vi "LabVIEW_2_Arduino_3D_Print_Fan_Zhu.vi"() -> ()   [LabVIEW 2017]
uses:
  <vilib>/Instr/_visa.llb/VISA Flush IO Buffer Mask.ctl
  <vilib>/Instr/_visa.llb/VISA Configure Serial Port (Instr).vi
panel:
  out "2nd buffer":string
  in  "VISA resource name 2":refnum<visa-resource-name>
  in  "baud rate (9600) 2":u32=9600
  in  "Turn on motor\n(Green = ON)":bool
  in  "Stop Motor":bool
  in  "VISA resource name":refnum<visa-resource-name>
  in  "baud rate (9600)":u32=9600
  out "Motor State":string
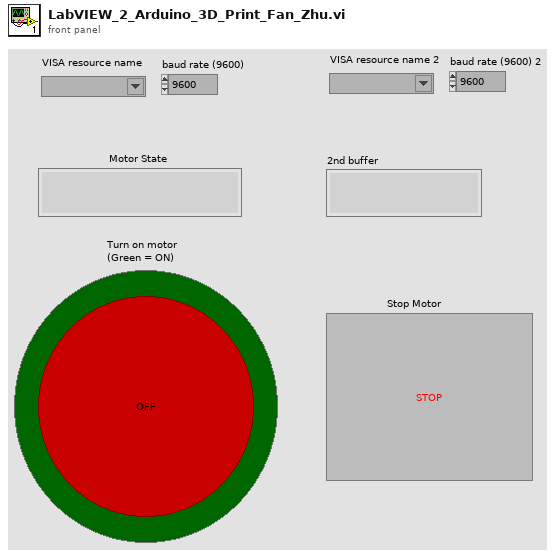
[diagram p1: front panel]
types:
  T1 = typedef "VISA Flush IO Buffer Mask.ctl" = u16
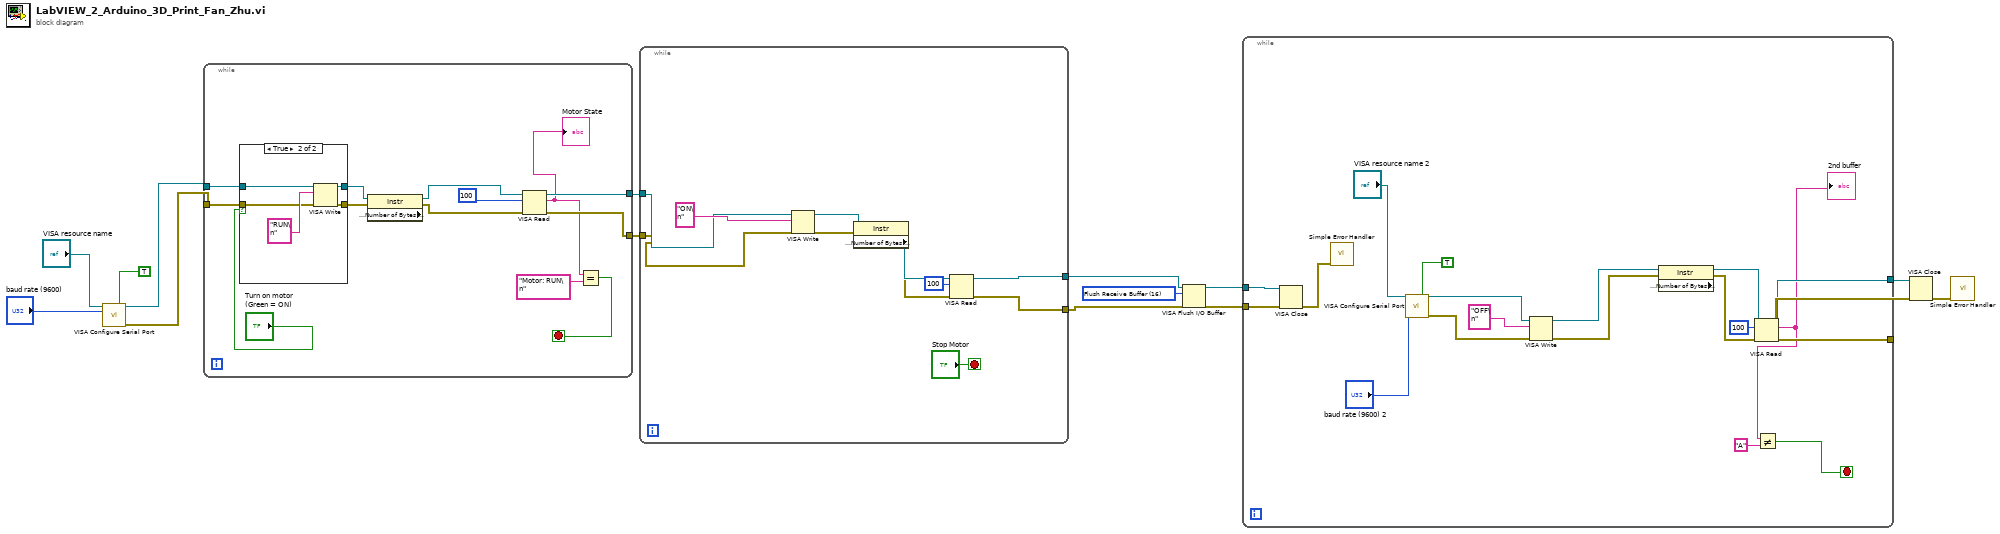
[diagram p0: block diagram]
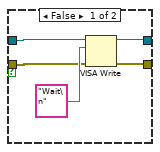
[diagram p2: hidden frame]
diagram:
  w3 = T1 16 items=["Flush Receive Buffer"=16, "Write Transmit Buffer to Device"=32, "Flush Receive Buffer (No I/O)"=64, "Flush Transmit Buffer"=128] ("Mask")
  n1 = call-poly "VISA Configure Serial Port"("VISA resource name"="VISA resource name", "Enable Termination\nChar (T)"=TRUE ("Enable Termination\nChar (T)"), "baud rate (9600)"="baud rate (9600)") -> ("VISA resource name out"=w13:refnum<visa-resource-name>, "error out"=w12:errorcluster)  [unwired: 11 in]
  n2 = while {
    tunnel: w13 -> [w25]
    tunnel: w12 -> [w24]
    tunnel: [w19] -> w11
    tunnel: [w18] -> w10
    stop <- w22 stop-if-true
    n3 = case shown="True" "Turn on motor\n(Green = ON)" {
      tunnel: [w29 w38] -> w27
      tunnel: [w30 w37] -> w26
      tunnel: w25 -> [w31 w35]
      tunnel: w24 -> [w32 w34]
      frame False {
        n4 = VISA Write(VISA resource name=w31, write buffer="Wait\n", error in (no error)=w32) -> (VISA resource name out=w30:refnum<visa-resource-name>, error out=w29:errorcluster)  [unwired: 1 out]
      }
      frame True {
        n5 = VISA Write(VISA resource name=w35, write buffer="RUN\n", error in (no error)=w34) -> (VISA resource name out=w37:refnum<visa-resource-name>, error out=w38:errorcluster)  [unwired: 1 out]
      }
    }
    n6 = property class="Instr" props=["Serial Settings:Number of Bytes at Serial Port"](reference=w26, error in=w27) -> (reference out=w21:refnum<visa-resource-name>, error out=w20:errorcluster)  [unwired: 1 out]
    n7 = VISA Read(VISA resource name=w21, byte count=u32 100, error in (no error)=w20) -> (VISA resource name out=w19:refnum<visa-resource-name>, read buffer=w16:string, error out=w18:errorcluster)  [unwired: 1 out]
    "Motor State" <- w16
    n8 = Equal?(x=w16, y="Motor: RUN\n") -> (x = y?=w22:bool)
  }
  n9 = while {
    tunnel: w11 -> [w41]
    tunnel: w10 -> [w40]
    tunnel: [w43] -> w5
    tunnel: [w42] -> w4
    stop <- "Stop Motor" stop-if-true
    n10 = VISA Write(VISA resource name=w41, write buffer="ON\n", error in (no error)=w40) -> (VISA resource name out=w44:refnum<visa-resource-name>, error out=w45:errorcluster)  [unwired: 1 out]
    n11 = property class="Instr" props=["Serial Settings:Number of Bytes at Serial Port"](reference=w44, error in=w45) -> (reference out=w49:refnum<visa-resource-name>, error out=w48:errorcluster)  [unwired: 1 out]
    n12 = VISA Read(VISA resource name=w49, byte count=u32 100, error in (no error)=w48) -> (VISA resource name out=w43:refnum<visa-resource-name>, error out=w42:errorcluster)  [unwired: 2 out]
  }
  n13 = VISA Flush I/O Buffer(VISA resource name=w5, mask (16)=w3, error in (no error)=w4) -> (VISA resource name out=w7:refnum<visa-resource-name>, error out=w6:errorcluster)
  n14 = while {
    tunnel: w7 -> [w66]
    tunnel: [w54] -> w9
    tunnel: w6 -> [w55]
    tunnel: [w53] -> w8
    stop <- w57 stop-if-true
    n15 = VISA Close(VISA resource name=w66, error in (no error)=w55) -> (error out=w67:errorcluster)
    n16 = call <vilib>:"Simple Error Handler.vi"("error in (no error)"=w67) -> ()  [unwired: 4 in, 5 out]
    n17 = call-poly "VISA Configure Serial Port"("VISA resource name"="VISA resource name 2", "Enable Termination\nChar (T)"=TRUE ("Enable Termination\nChar (T)"), "baud rate (9600)"="baud rate (9600) 2") -> ("VISA resource name out"=w64:refnum<visa-resource-name>, "error out"=w63:errorcluster)  [unwired: 11 in]
    n18 = VISA Write(VISA resource name=w64, write buffer="OFF\n", error in (no error)=w63) -> (VISA resource name out=w59:refnum<visa-resource-name>, error out=w58:errorcluster)  [unwired: 1 out]
    n19 = property class="Instr" props=["Serial Settings:Number of Bytes at Serial Port"](reference=w59, error in=w58) -> (reference out=w62:refnum<visa-resource-name>, error out=w61:errorcluster)  [unwired: 1 out]
    n20 = VISA Read(VISA resource name=w62, byte count=u32 100, error in (no error)=w61) -> (VISA resource name out=w54:refnum<visa-resource-name>, read buffer=w52:string, error out=w53:errorcluster)  [unwired: 1 out]
    "2nd buffer" <- w52
    n21 = Not Equal?(x=w52, y="A") -> (x != y?=w57:bool)
  }
  n22 = VISA Close(VISA resource name=w9, error in (no error)=w8) -> (error out=w14:errorcluster)
  n23 = call <vilib>:"Simple Error Handler.vi"("error in (no error)"=w14) -> ()  [unwired: 4 in, 5 out]
